vi "Change Mixer Speed.vi"(8 "error in (no error)":errorcluster, 10 "Mixer":dbl(ring) items=["0%"=0.075, "25%"=0.08, "50%"=0.085, "75%"=0.09, "100%"=0.095], 11 "Feeder Actor.lvlib:Mixer.lvclass":refnum<class "Mixer.lvclass">) -> (0 "error out":errorcluster, 3 "Actor out":refnum<class "Actor.lvclass">)   [LabVIEW 2018, in "Feeder Actor.lvlib" / "Mixer.lvclass"]
uses:
  Mixer.lvclass
  <vilib>/ActorFramework/Actor/Actor.lvclass
  C:/Program Files/National Instruments/LabVIEW 2018/vi.lib/ActorFramework/Actor/Actor.lvclass
  Mixer.lvclass/Mixer.ctl
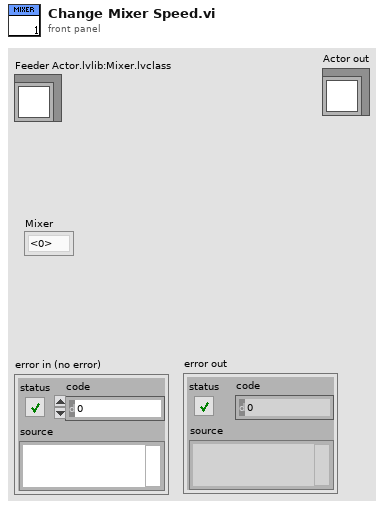
[diagram p1: front panel]
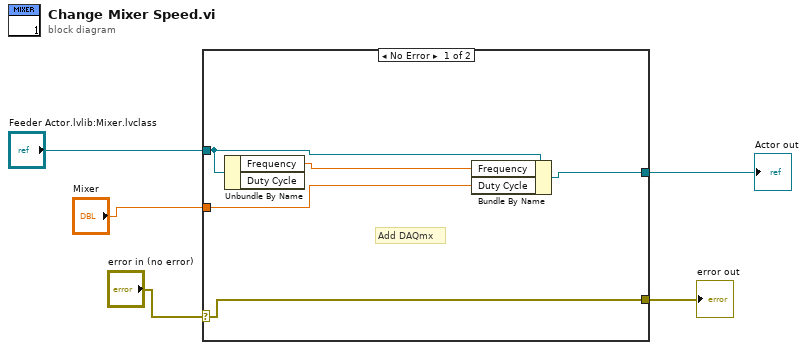
[diagram p0: block diagram]
diagram:
  n1 = case shown="No Error" "error in (no error)" {
    selector: "error in (no error)" -> [w8 w11]
    tunnel: "Feeder Actor.lvlib:Mixer.lvclass" -> [w9 w12]
    tunnel: [w10 w12] -> w4
    tunnel: [w8 w11] -> w2
    tunnel: "Mixer" -> [w6 _]
    frame No Error {
      # "Add DAQmx"
      n2 = Unbundle By Name(w9) -> ("Frequency"=w7:dbl)  [unwired: 1 out]
      n3 = Bundle By Name(cluster=w9, "Frequency"=w7, "Duty Cycle"=w6) -> (w10:refnum<class "Mixer.lvclass">)
    }
    frame Error {
    }
  }
  "Actor out" <- w4
  "error out" <- w2
